vi "Main.vi"(11 "Module Admin":refnum<class "Delacor_lib_QMH_Module Admin.lvclass">) -> ()   [LabVIEW 2024, in "Hardware Controller.lvlib"]
doc: "This template is based off of the Queued Message Handler design pattern and the Queued Message Handler project template that ships with LabVIEW.\n\nThe main difference is that the queue is private to this module and communication between modules is performed via Broadcast and Request events.\n\nRequest events are wrapped in public API methods and are handled in the Event Handling Loop (EHL) of this VI. Any module can register for Broadcast events sent by this module. The EHL generates messages based on user interface actions.\n\nThe Message Handling Loop (MHL) processes messages generated by the EHL, or by other messages. The messages are string values, so new messages can be added easily to the Message Cases case structure in the MHL. Each message cluster can also provide an optional value for Message Data, which is a variant that can be converted to whatever message-specific data is required.\n_____\nBased on DQMH Project Template 7.0.0.1280."
uses:
  Hardware Controller.lvlib
  <vilib>/Delacor/Delacor QMH/Libraries/Module Admin_class/Delacor_lib_QMH_Module Admin.lvclass
  Module Data--cluster.ctl
  <vilib>/Delacor/Delacor QMH/Libraries/Message Queue_class/Delacor_lib_QMH_Message Queue.lvclass/Delacor_lib_QMH_Message Queue.ctl
  Stop Argument--cluster.ctl
  <vilib>/Delacor/Delacor QMH/Libraries/Module Admin_class/Delacor_lib_QMH_Module Admin.lvclass/Delacor_lib_QMH_Module Admin.ctl
  <vilib>/Utility/miscctls.llb/LVPointTypeDef.ctl
  <vilib>/Delacor/Delacor QMH/Libraries/Message Queue_class/Delacor_lib_QMH_Enqueue Message (Single).vi
  <vilib>/Delacor/Delacor QMH/Libraries/Module Admin_class/Delacor_lib_QMH_Get External Launch.vi
  <vilib>/Delacor/Delacor QMH/Libraries/Message Queue_class/Delacor_lib_QMH_Message Queue.lvclass
panel:
  out "System State":map{string, dbl}(c390)
  out "error out":errorcluster
  out "Status":string
  in  "Simulate MHL Error":bool
  in  "Simulate EHL Error":bool
  # "This template is for the DQMH framework. See the block diagram for more information on how to use this template."
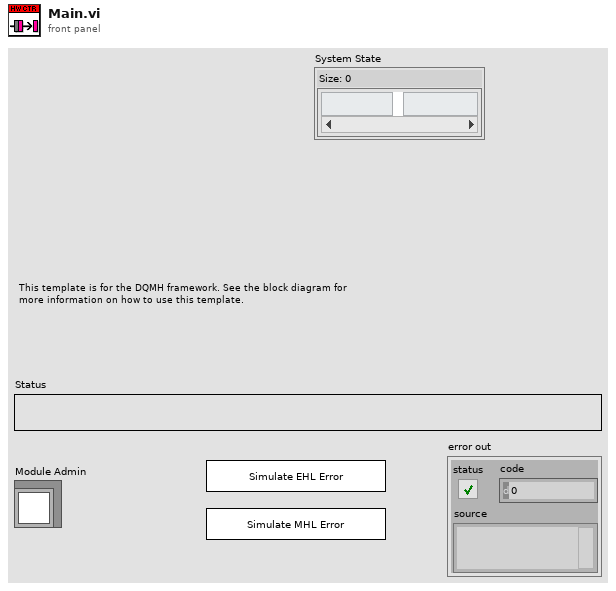
[diagram p1: front panel]
types:
  T1 = typedef "Hardware Controller.lvlib/Request Events--cluster.ctl" = cluster{"Stop Module":refnum<user-event>, "Show Panel":refnum<user-event>, "Hide Panel":refnum<user-event>, "Get Module Execution Status":refnum<user-event>, "Show Diagram":refnum<user-event>, "Private":cluster{"Start System State Broadcast Helper Loop":refnum<user-event>}}
  T2 = typedef "Hardware Controller.lvlib/Module Data--cluster.ctl" = cluster{"Status":string, "System State":map{string, dbl}}
  T3 = enum32{"invalid lock state", "Not Locked", "Locked (No Password)", "Password-protected"}
  T4 = typedef "Hardware Controller.lvlib/Stop Argument--cluster.ctl" = cluster{"Origin":string, "Exit via Stop Module Req?":bool, "Wait for Module to stop?":bool}
  T5 = typedef "LVPointTypeDef.ctl" = cluster{"Horizontal":i16, "Vertical":i16}
  T6 = enum32{"Invalid", "Standard", "Closed", "Hidden", "Minimized", "Maximized"}
  T7 = typedef "EtherCAT Configuration.ctl" = cluster{"ENI File":path, "Drives":cluster{"Drive Key":string, "Read Variables":cluster{"Name":string, "Index":u16, "Bit":u8, "Type":string}[], "Write Variables":cluster{"Name":string, "Index":u16}[]}[]}
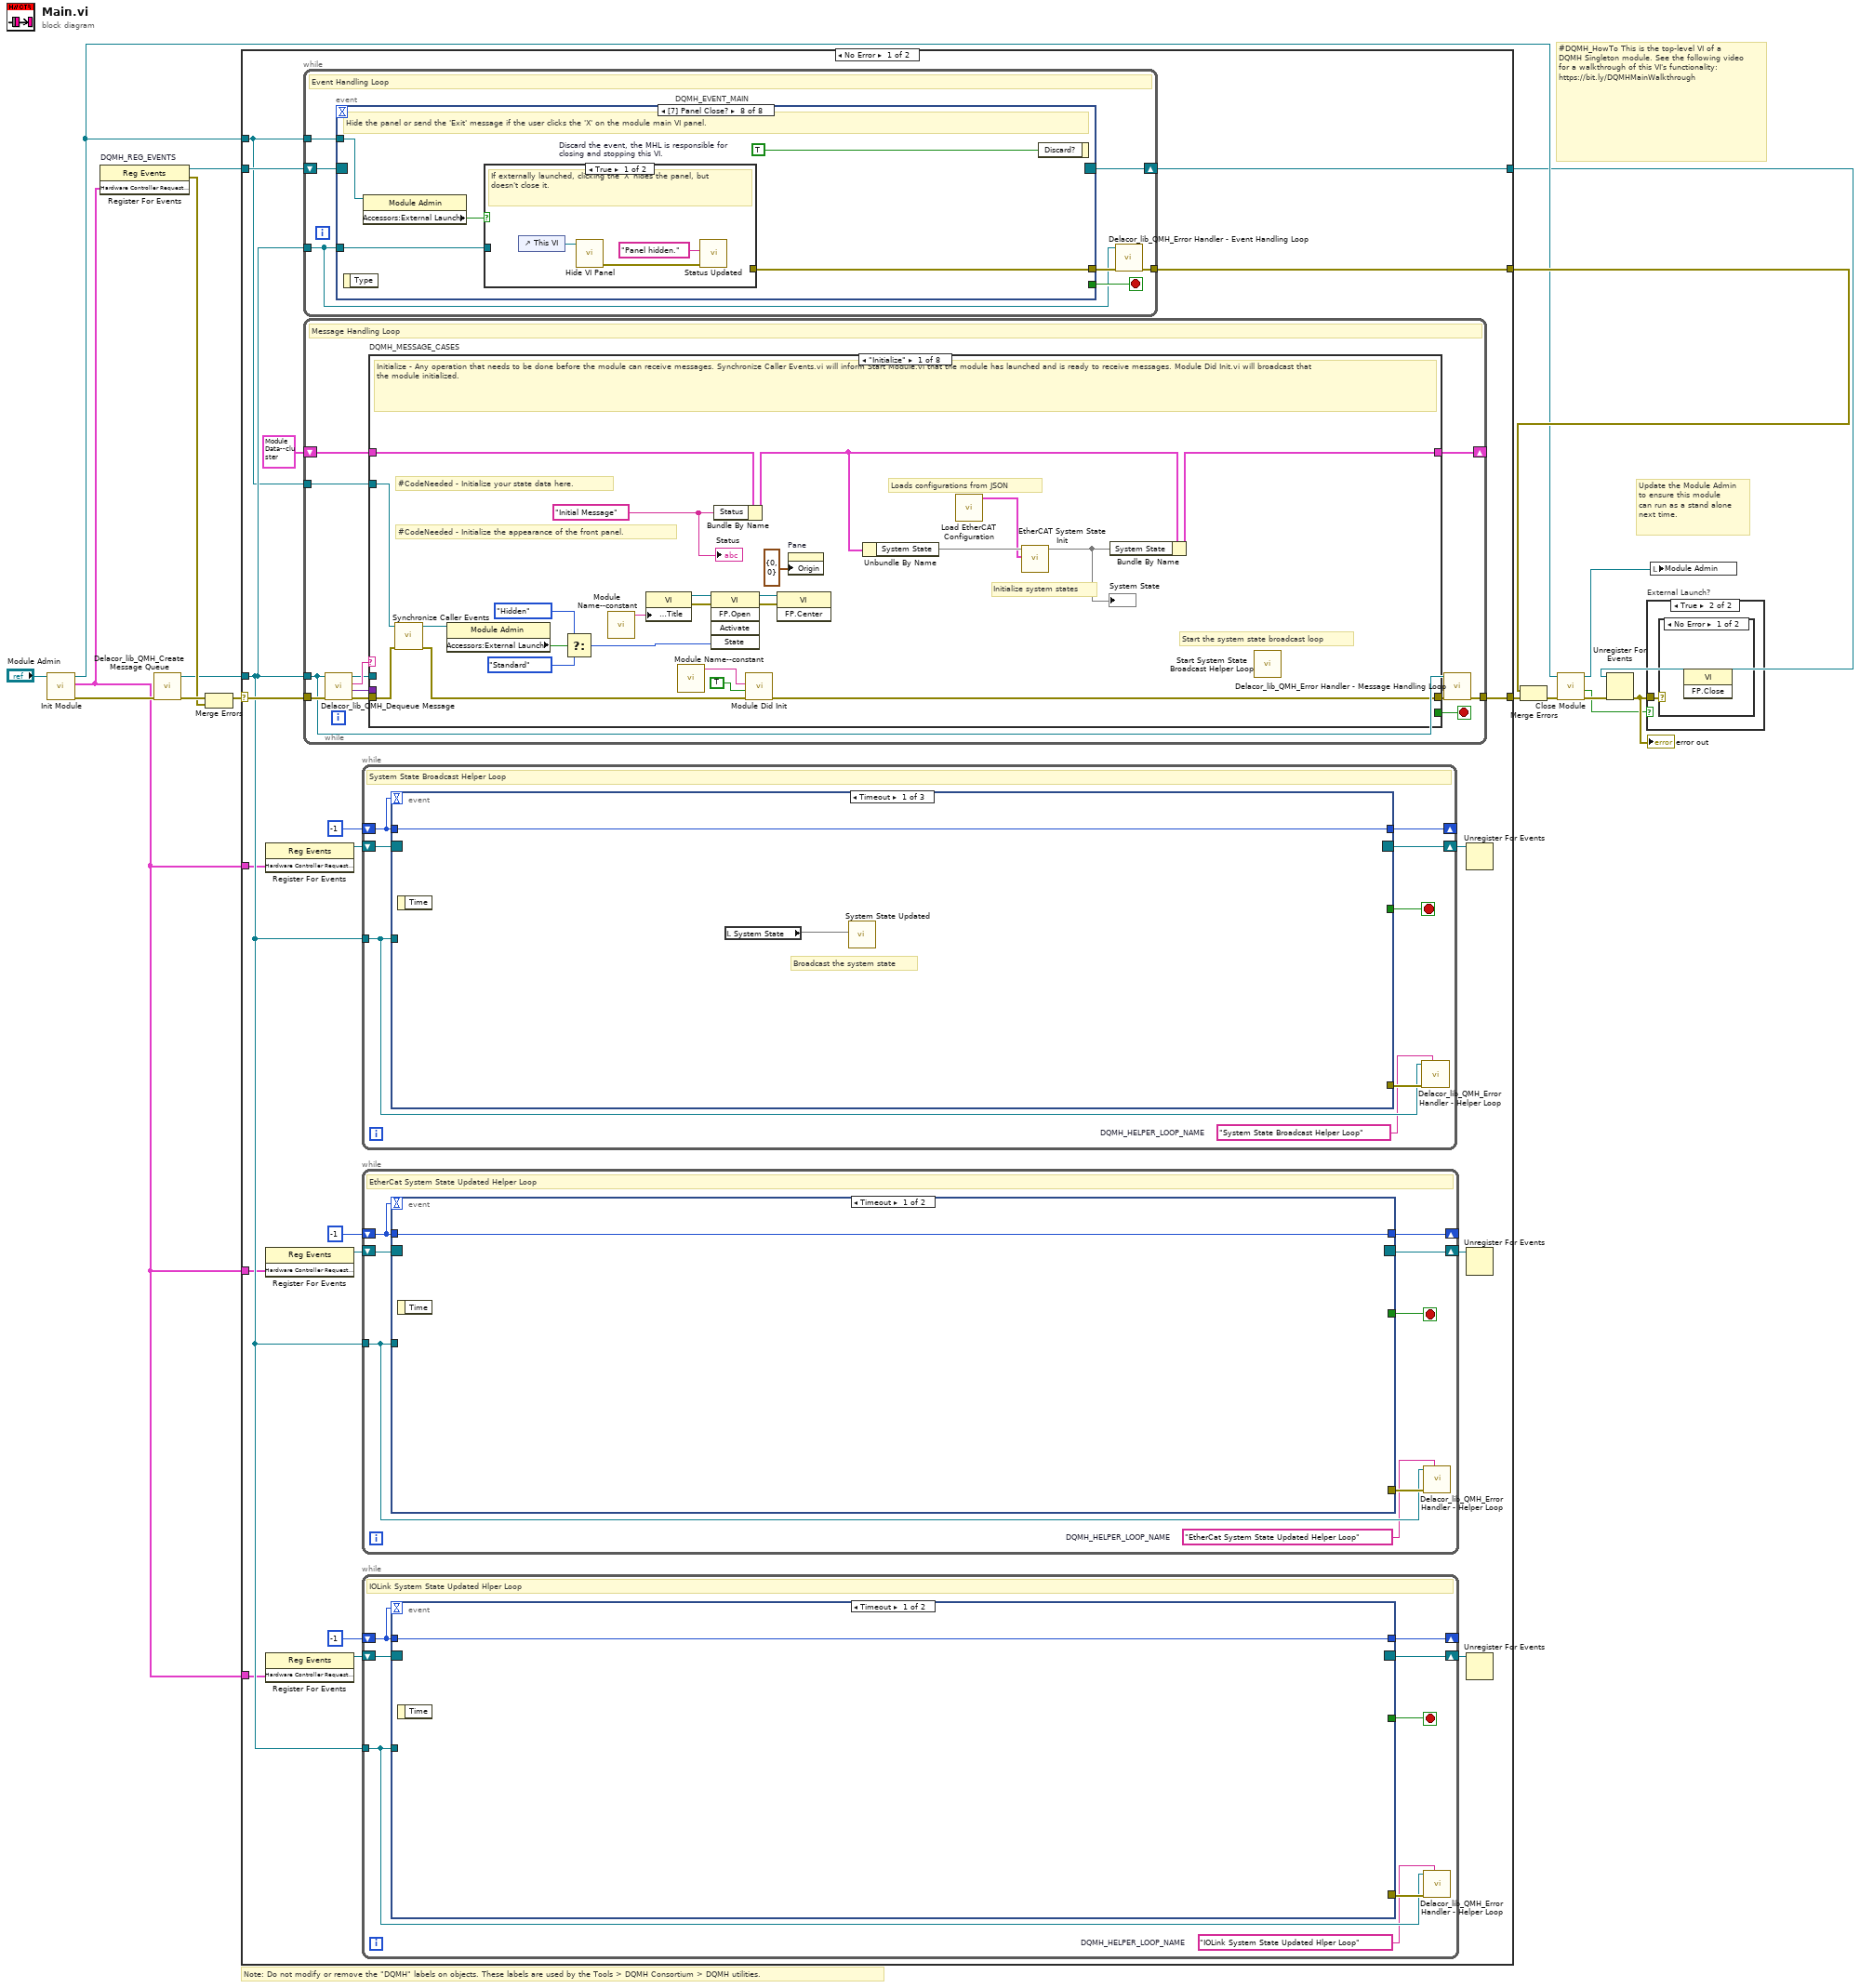
[diagram p0: block diagram]
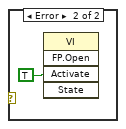
[diagram p3: hidden frame]
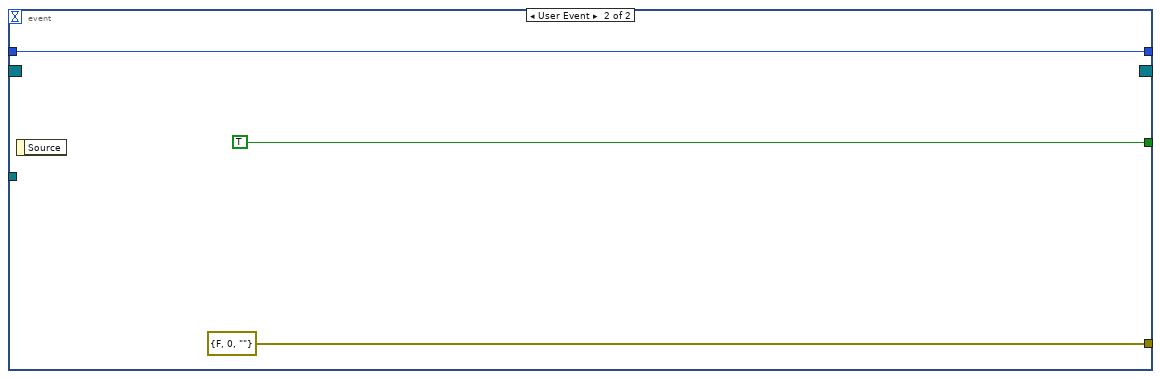
[diagram p4: hidden frame]
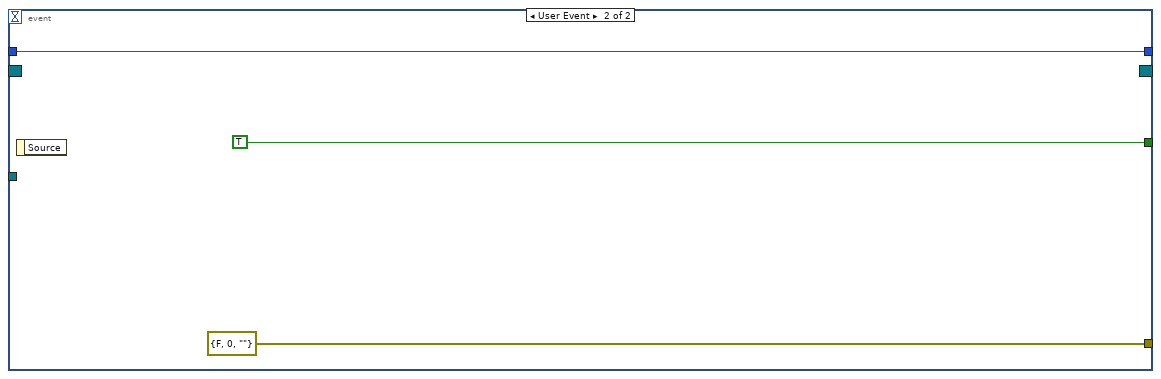
[diagram p5: hidden frame]
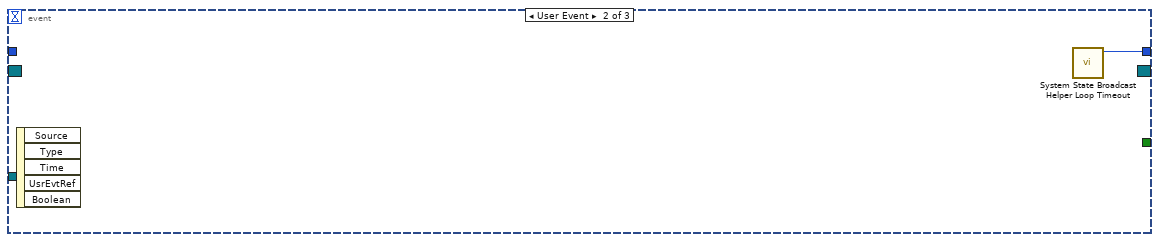
[diagram p6: hidden frame]
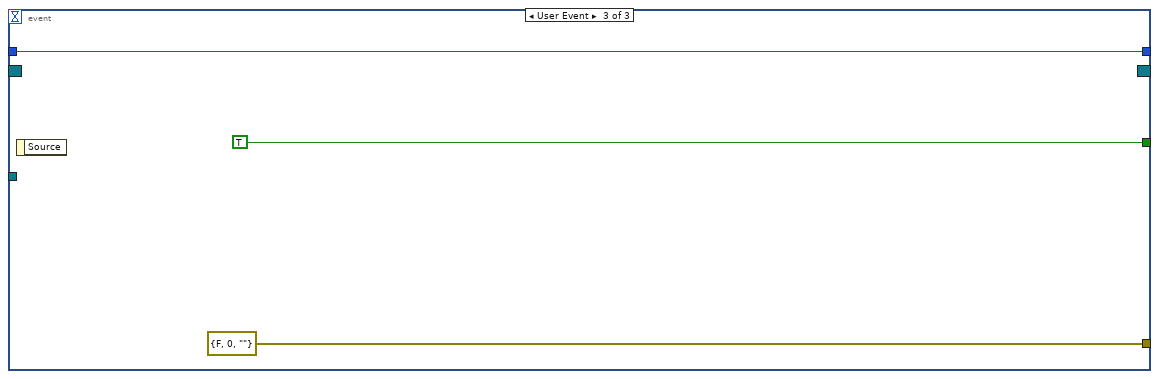
[diagram p7: hidden frame]
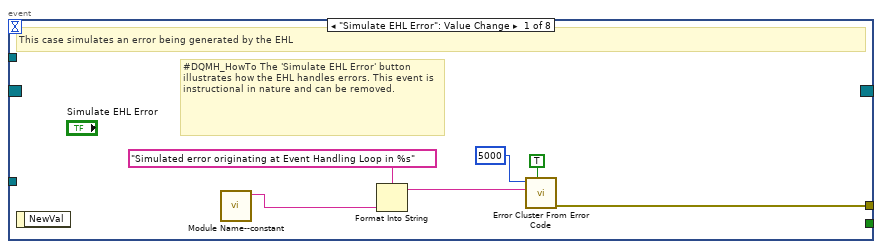
[diagram p8: hidden frame]
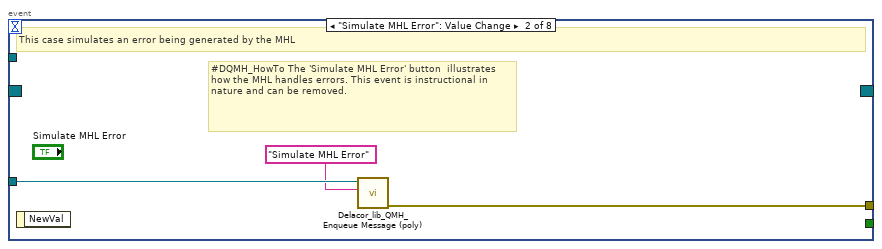
[diagram p9: hidden frame]
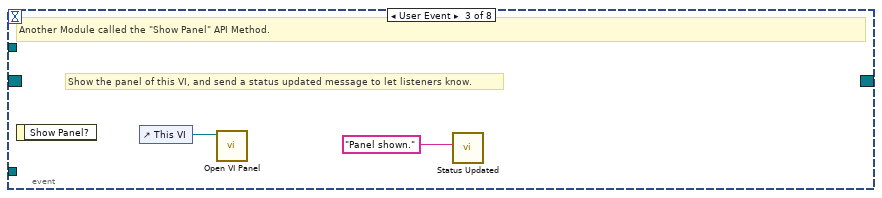
[diagram p10: hidden frame]
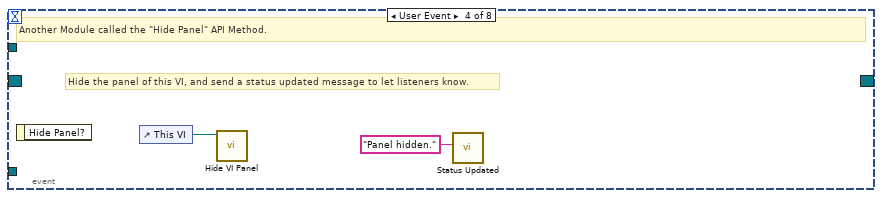
[diagram p11: hidden frame]
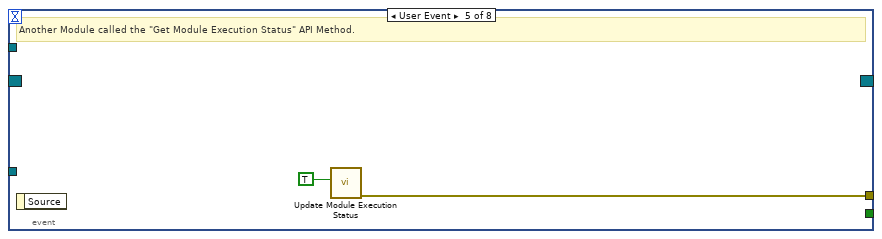
[diagram p12: hidden frame]
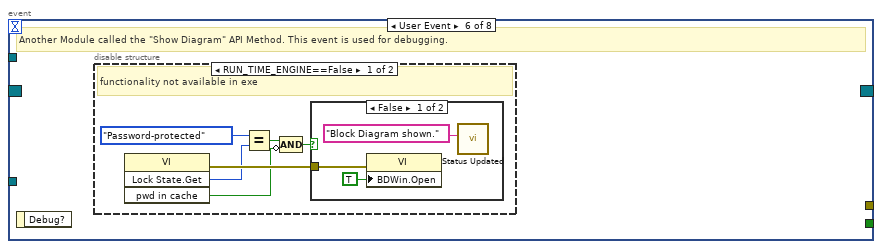
[diagram p13: hidden frame]
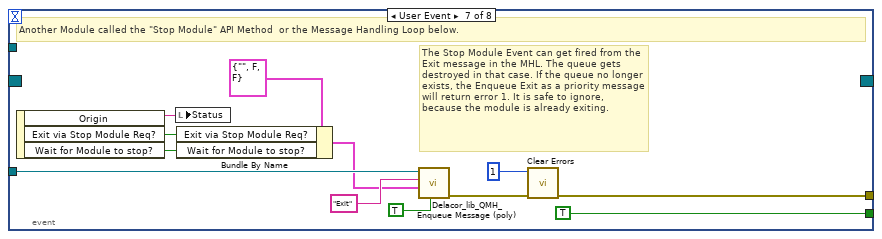
[diagram p16: hidden frame]
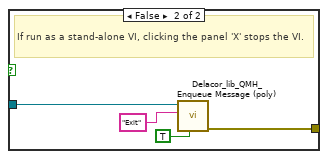
[diagram p17: hidden frame]
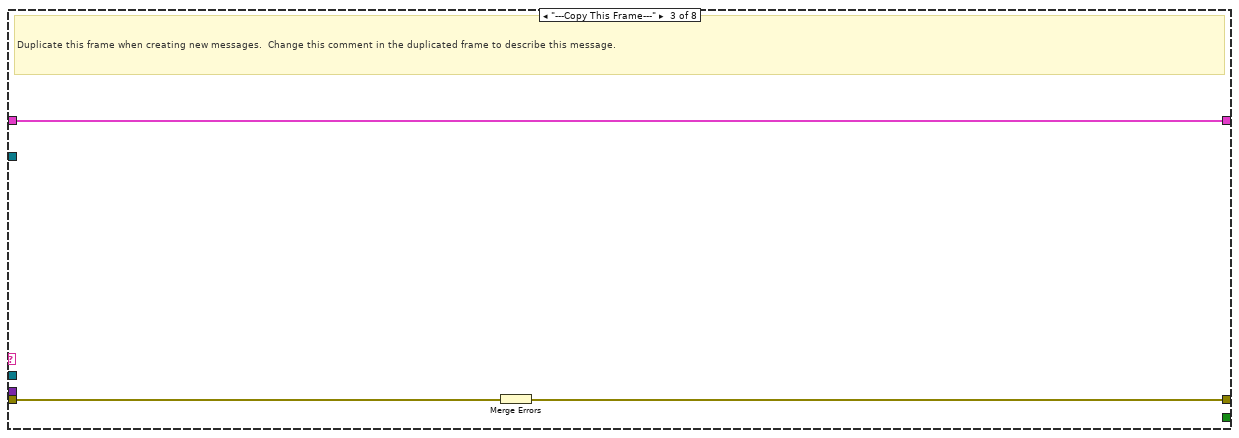
[diagram p19: hidden frame]
diagram:
  # "#DQMH_HowTo This is the top-level VI of a DQMH Singleton module. See the following video for a walkthrough of this VI's functionality: https://bit.ly/DQMHMainWalkthrough"
  # "Note: Do not modify or remove the \"DQMH\" labels on objects. These labels are used by the Tools > DQMH Consortium > DQMH utilities."
  # "Update the Module Admin to ensure this module can run as a stand alone next time."
  n1 = call "Init Module.vi"("Singleton Module Admin in"="Module Admin") -> ("error out"=w16:errorcluster, "Hardware Controller Request Events"=w1:T1, "Singleton Module Admin out"=w8:refnum<class "Delacor_lib_QMH_Module Admin.lvclass">)  [unwired: 8 in]
  n2 = register-events "DQMH_REG_EVENTS"(w1) -> (reference out=w6:refnum<event-registration>, error out=w9:errorcluster)  [unwired: 2 in]
  n3 = call <vilib>:"Delacor_lib_QMH_Create Message Queue.vi"("error in"=w16) -> ("error out"=w11:errorcluster, "Message Queue"=w5:refnum<class "Delacor_lib_QMH_Message Queue.lvclass">)  [unwired: 9 in]
  n4 = Merge Errors(w11, w9) -> (w10:errorcluster)
  n5 = case shown="No Error" w10 {
    selector: w10 -> [w35 w232]
    tunnel: [w37 w231] -> w17
    tunnel: [w34 w230] -> w7
    tunnel: w6 -> [w32 w230]
    tunnel: w5 -> [w31 w225]
    tunnel: [w36 _] -> w14
    tunnel: w8 -> [w30 w226]
    tunnel: w1 -> [w29 _]
    tunnel: w1 -> [w25 _]
    tunnel: w1 -> [w21 _]
    frame No Error {
      n6 = register-events ("DQMH_HELPER_REGFOREVENTS")(w29) -> (reference out=w27:refnum<event-registration>)  [unwired: 2 in, 1 out]
      n7 = register-events ("DQMH_HELPER_REGFOREVENTS")(w25) -> (reference out=w23:refnum<event-registration>)  [unwired: 2 in, 1 out]
      n8 = register-events ("DQMH_HELPER_REGFOREVENTS")(w21) -> (reference out=w19:refnum<event-registration>)  [unwired: 2 in, 1 out]
      n9 = while {
        tunnel: w31 -> [w76]
        shift-right: [w79] -> w34
        shift-left: w32 -> [w80]
        tunnel: [w81] -> w36
        tunnel: w30 -> [w77]
        stop <- w78 stop-if-true
        # "Event Handling Loop"
        n10 = event "DQMH_EVENT_MAIN" shown="[7] Panel Close?" {
          selector: w80 -> [_ _ _ _ _ _ _ _]
          dyn-events: [_ _ _ _ _ _ _ _] -> w79
          timeout: _ -> [_ _ _ _ _ _ _ _]
          tunnel: [_ _ _ _ _ _ TRUE ("Discard?") _] -> w78
          tunnel: w76 -> [_ w90 _ _ _ _ w114 w121]
          tunnel: [w88 w91 _ _ w97 _ w117 w123] -> w82
          tunnel: w77 -> [_ _ _ _ _ _ _ w120]
          event "Simulate EHL Error": Value Change {
            # "#DQMH_HowTo The 'Simulate EHL Error' button  illustrates how the EHL handles errors. This event is instructional in nature and can be removed."
            # "This case simulates an error being generated by the EHL"
            n11 = event-data() -> ()  [unwired: 1 in, 1 out]
            n12 = call "Module Name--constant.vi"() -> ("Module Name"=w85:string)  [unwired: 11 in]
            n13 = Format Into String(format string="Simulated error originating at Event Handling Loop in %s", w85) -> (resulting string=w86:string)  [unwired: 2 in, 1 out]
            n14 = call <vilib>:"Error Cluster From Error Code.vi"("show call chain? (False)"=TRUE, "error message (\"\")"=w86, "error code (0)"=5000) -> ("error out"=w88:errorcluster)  [unwired: 6 in]
          }
          event "Simulate MHL Error": Value Change {
            # "#DQMH_HowTo The 'Simulate MHL Error' button  illustrates how the MHL handles errors. This event is instructional in nature and can be removed."
            # "This case simulates an error being generated by the MHL"
            n15 = event-data() -> ()  [unwired: 1 in, 1 out]
            n16 = call-poly <vilib>:"Delacor_lib_QMH_Enqueue Message (poly).vi"("Message"="Simulate MHL Error", "Message Queue in"=w90) -> ("error out"=w91:errorcluster)  [unwired: 8 in, 1 out]
          }
          event User Event {
            # "Show the panel of this VI, and send a status updated message to let listeners know."
            # "Another Module called the \"Show Panel\" API Method."
            n17 = event-data() -> ()  [unwired: 1 in, 1 out]
            n18 = control-ref of="This VI"() -> (w93:refnum<vi>)
            n19 = call "Open VI Panel.vi"("VI"=w93) -> ()  [unwired: 10 in, 1 out]
            n20 = call "Status Updated.vi"("Status"="Panel shown." ("format string")) -> ()  [unwired: 10 in, 1 out]
          }
          event User Event {
            # "Hide the panel of this VI, and send a status updated message to let listeners know."
            # "Another Module called the \"Hide Panel\" API Method."
            n21 = event-data() -> ()  [unwired: 1 in, 1 out]
            n22 = control-ref of="This VI"() -> (w95:refnum<vi>)
            n23 = call "Hide VI Panel.vi"("VI"=w95) -> ()  [unwired: 10 in, 1 out]
            n24 = call "Status Updated.vi"("Status"="Panel hidden." ("format string")) -> ()  [unwired: 10 in, 1 out]
          }
          event User Event {
            # "Another Module called the \"Get Module Execution Status\" API Method."
            n25 = event-data() -> ()  [unwired: 1 in, 1 out]
            n26 = call "Update Module Execution Status.vi"("Running?"=TRUE) -> ("error out"=w97:errorcluster)  [unwired: 10 in]
          }
          event User Event {
            # "Another Module called the \"Show Diagram\" API Method. This event is used for debugging."
            n27 = event-data() -> ()  [unwired: 1 in, 1 out]
            n28 = disable-structure shown="RUN_TIME_ENGINE==False" {
              frame condition #0 (active) {
                # "functionality not available in exe"
                n29 = invoke class="VI" method="Lock State.Get"() -> (error out=w103:errorcluster, "Get Lock State"=w102:T3, "pwd in cache"=w99:bool)  [unwired: 4 in, 1 out]
                n30 = Equal?(x=T3."Password-protected", y=w102) -> (x = y?=w100:bool)
                n31 = Compound Arithmetic op=AND(w100, invert w99) -> (w98:bool)
                n32 = case shown="False" w98 {
                  tunnel: w103 -> [w106 _]
                  frame False {
                    n33 = property class="VI"(error in=w106, "BDWin.Open"=TRUE ("Block Diagram Window:Open")) -> ()  [unwired: 1 in, 2 out]
                    n34 = call "Status Updated.vi"("Status"="Block Diagram shown." ("format string")) -> ()  [unwired: 10 in, 1 out]
                  }
                  frame True {
                    # "Password-protected VI, and the password is not in the cache. Do not show the diagram."
                  }
                }
              }
              frame condition #1 {
              }
            }
          }
          event User Event {
            # "The Stop Module Event can get fired from the Exit message in the MHL. The queue gets destroyed in that case. If the queue no longer exists, the Enqueue Exit as a priority message will return error 1. It is safe to ignore, because the module is already exiting."
            # "Another Module called the \"Stop Module\" API Method  or the Message Handling Loop below."
            n35 = event-data() -> ("Origin"=w113:string, "Exit via Stop Module Req?"=w109:bool, "Wait for Module to stop?"=w108:bool)  [unwired: 1 in]
            n36 = local write "Status"(w113) -> ()
            n37 = Bundle By Name(cluster=T4 {"Origin"="", "Exit via Stop Module Req?"=FALSE, "Wait for Module to stop?"=FALSE} ("Stop Argument"), "Exit via Stop Module Req?"=w109, "Wait for Module to stop?"=w108) -> (w107:T4)
            n38 = call-poly <vilib>:"Delacor_lib_QMH_Enqueue Message (poly).vi"("Priority Message? (F)"=TRUE, "Message Data"=w107, "Message"="Exit", "Message Queue in"=w114) -> ("error out"=w118:errorcluster)  [unwired: 6 in, 1 out]
            n39 = call <vilib>:"Clear Errors.vi"("error in (no error)"=w118, "specific error code to clear (0: all)"=1) -> ("error out"=w117:errorcluster)  [unwired: 4 in, 1 out]
          }
          event Panel Close? {
            w122 = TRUE  # Discard the event, the MHL is responsible for closing and stopping this VI.
            # "Hide the panel or send the 'Exit' message if the user clicks the 'X' on the module main VI panel."
            n40 = event-data() -> ()  [unwired: 1 in, 1 out]
            n41 = property class="Module Admin"(reference=w120) -> ("Accessors:External Launch"=w119:bool)  [unwired: 1 in, 2 out]
            n42 = case shown="True" w119 {
              tunnel: w121 -> [_ w129]
              tunnel: [_ w130] -> w123
              frame True {
                # "If externally launched, clicking the 'X' hides the panel, but doesn't close it."
                n43 = control-ref of="This VI"() -> (w126:refnum<vi>)
                n44 = call "Hide VI Panel.vi"("VI"=w126) -> ("error out"=w124:errorcluster)  [unwired: 10 in]
                n45 = call "Status Updated.vi"("error in"=w124, "Status"="Panel hidden." ("format string")) -> ()  [unwired: 9 in, 1 out]
              }
              frame False {
                # "If run as a stand-alone VI, clicking the panel 'X' stops the VI."
                n46 = call-poly <vilib>:"Delacor_lib_QMH_Enqueue Message (poly).vi"("Priority Message? (F)"=TRUE, "Message"="Exit", "Message Queue in"=w129) -> ("error out"=w130:errorcluster)  [unwired: 7 in, 1 out]
              }
            }
            n47 = event-data("Discard?"=w122) -> ()  [unwired: 1 in, 1 out]
          }
        }
        n48 = call-dynamic "Delacor_lib_QMH_Error Handler - Event Handling Loop.vi"("error in"=w82, "Message Queue in"=w76) -> ("dup error in"=w81:errorcluster)  [unwired: 8 in, 1 out]
      }
      n49 = while {
        tunnel: w31 -> [w131]
        shift-right: [w137] -> _
        shift-left: T2 {"Status"="", "System State"={}} ("Data Cluster") -> [w138]
        tunnel: w35 -> [w141]
        tunnel: [w139] -> w37
        tunnel: w30 -> [w132]
        stop <- w136 stop-if-true
        # "Message Handling Loop"
        n50 = call-dynamic "Delacor_lib_QMH_Dequeue Message.vi"("error in"=w141, "Message Queue in"=w131) -> ("error out"=w140:errorcluster, "Message Data"=w134:variant, "Message"=w135:string, "Message Queue out"=w133:refnum<class "Delacor_lib_QMH_Message Queue.lvclass">)  [unwired: 6 in]
        n51 = case "DQMH_MESSAGE_CASES" shown="\"Initialize\"" w135 {
          selector: w135 -> [_ _ _ _ _ _ _ w220]
          tunnel: w133 -> [_ _ _ _ _ w186 w208 _]
          tunnel: w140 -> [w164 w168 w171 w173 w182 w193 w214 w223]
          tunnel: [w162 w168 w170 w173 w181 w189 w209 w224] -> w142
          tunnel: w138 -> [w153 w167 w169 w172 w179 w188 w207 w221]
          tunnel: [w144 w167 w169 w172 w179 w188 w207 w221] -> w137
          tunnel: [_ _ _ _ _ _ w206 _] -> w136
          tunnel: w134 -> [_ _ _ _ _ w187 w205 _]
          tunnel: w132 -> [w154 _ _ _ _ w185 w200 _]
          frame "Initialize" {
            w149 = "Initial Message" ("Initial Message")
            # "Start the system state broadcast loop"
            # "Initialize system states"
            # "Loads configurations from JSON"
            # "#CodeNeeded - Initialize the appearance of the front panel."
            # "#CodeNeeded - Initialize your state data here."
            # "Initialize - Any operation that needs to be done before the module can receive messages. Synchronize Caller Events.vi will inform Start Module.vi that the module has launched and is ready to receive messages. Module Did Init.vi will broadcast that the module initialized."
            n52 = call "Synchronize Caller Events.vi"("error in"=w164, "Singleton Module Admin in"=w154) -> ("error out"=w163:errorcluster, "Singleton Module Admin out"=w150:refnum<class "Delacor_lib_QMH_Module Admin.lvclass">)  [unwired: 8 in]
            n53 = property class="Module Admin"(reference=w150) -> ("Accessors:External Launch"=w158:bool)  [unwired: 1 in, 2 out]
            n54 = Select(t=T6."Hidden" ("State"), s=w158, f=T6."Standard" ("State")) -> (s? t:f=w155:T6)
            n55 = call "Module Name--constant.vi"() -> ("Module Name"=w161:string)  [unwired: 11 in]
            n56 = property class="VI"("Front Panel.Title"=w161) -> (reference out=w160:refnum<vi>, error out=w166:errorcluster)  [unwired: 2 in]
            n57 = call "Module Name--constant.vi"() -> ("Module Name"=w151:string)  [unwired: 11 in]
            n58 = invoke class="VI" method="FP.Open"(reference=w160, error in=w166, "State"=w155) -> (reference out=w159:refnum<vi>, error out=w165:errorcluster)  [unwired: 2 in, 3 out]
            n59 = Bundle By Name(cluster=w153, "Status"=w149) -> (w147:T2)
            n60 = call "Module Did Init.vi"("error in"=w163, "Initialized?"=TRUE, "Origin"=w151) -> ("error out"=w162:errorcluster)  [unwired: 8 in]
            n61 = invoke class="VI" method="FP.Center"(reference=w159, error in=w165) -> ()  [unwired: 1 in, 3 out]
            n62 = property on="Pane" class="Pane"("Origin"=T5 {"Horizontal"=0, "Vertical"=0}) -> ()  [unwired: 2 in, 2 out]
            n63 = Unbundle By Name(w147) -> ("System State"=w146:map{string, dbl})
            n64 = call "Load EtherCAT Configuration.vi"() -> ("Setup"=w145:T7)  [unwired: 11 in]
            n65 = call "EtherCAT System State Init.vi"("Setup"=w145, "System State"=w146) -> ("System State Out"=w143:map{string, dbl})  [unwired: 9 in]
            "System State" <- w143
            n66 = Bundle By Name(cluster=w147, "System State"=w143) -> (w144:T2)
            n67 = call "Start System State Broadcast Helper Loop.vi"() -> ()  [unwired: 11 in, 1 out]
            "Status" <- w149
          }
          frame "---Module Specific---" {
            # "Separator -- The following cases handle messages specific to this Module."
          }
          frame "---Copy This Frame---" {
            # "Duplicate this frame when creating new messages.  Change this comment in the duplicated frame to describe this message."
            n68 = Merge Errors(w171) -> (w170:errorcluster)
          }
          frame "---Exit and Error Handling---" {
            # "Separator - The following cases handle errors and exit messages."
          }
          frame "Simulate MHL Error" {
            # "#DQMH_HowTo The 'Simulate MHL Error' button  illustrates how the MHL handles errors. This event is instructional in nature and can be removed."
            # "Simulate an error occurring at the MHL"
            n69 = call "Module Name--constant.vi"() -> ("Module Name"=w175:string)  [unwired: 11 in]
            n70 = Format Into String(format string="Simulated error originating at Message Handling Loop in %s", w175) -> (resulting string=w176:string)  [unwired: 2 in, 1 out]
            n71 = call <vilib>:"Error Cluster From Error Code.vi"("show call chain? (False)"=TRUE, "error message (\"\")"=w176, "error code (0)"=5001) -> ("error out"=w180:errorcluster)  [unwired: 6 in]
            n72 = Merge Errors(w182, w180) -> (w181:errorcluster)
          }
          frame "Error" {
            # "#CodeRecommended - If the module is running in standalone mode (External Launch = FALSE), this code will pop up an error dialog and call the 'Exit' message if an error occurs. Add more fine-grained error management here."
            # "Error - Check the error message data and respond accordingly. This message is sent by the \"Error Handler\" VIs at the end of each loop in this application."
            n73 = property class="Module Admin"(reference=w185) -> ("Accessors:External Launch"=w184:bool)  [unwired: 1 in, 2 out]
            n74 = Variant To Data(error in=w193, type=errorcluster {"status"=FALSE, "code"=0, "source"=""} ("error constant"), Variant=w187) -> (data=w183:errorcluster, error out=w191:errorcluster)
            n75 = local write "error out"(w183) -> ()
            n76 = call "Error Reported.vi"("Error"=w183) -> ()  [unwired: 10 in, 1 out]
            n77 = case shown="False" w184 {
              tunnel: [w198 _] -> w190
              tunnel: w186 -> [w196 _]
              tunnel: w183 -> [w197 _]
              frame False {
                n78 = disable-structure shown="Default" {
                  disable-tunnel: w197 -> [w199 _]
                  frame condition #0 (active) {
                    # "If the module is running standalone, then pop up an error dialog and call the \"Exit\" message."
                    n79 = call <vilib>:"Simple Error Handler.vi"("error in (no error)"=w199) -> ()  [unwired: 4 in, 5 out]
                  }
                  frame condition #1 {
                    # "To prevent the Simple Error Handler VI from being loaded (e.g. when deploying to a Real-Time target), add the Conditional Disable Symbol \"DQMH_Disable_SEH\" to your project and set it to TRUE."
                  }
                }
                n80 = call-poly <vilib>:"Delacor_lib_QMH_Enqueue Message (poly).vi"("Priority Message? (F)"=TRUE, "Message"="Exit", "Message Queue in"=w196) -> ("error out"=w198:errorcluster)  [unwired: 7 in, 1 out]
              }
              frame True {
                # "If the module was launched externally, calling the Error Reported broadcast VI is the only action performed by the \"Error\" message. The module's caller can then process the error appropriately."
              }
            }
            n81 = Merge Errors(w191, w190) -> (w189:errorcluster)
          }
          frame "Exit" {
            w204 = 91  # 91: not all Exit messages will have an argument
            w206 = TRUE  # Stop the VI
            # "Release the message queue reference"
            # "#CodeNeeded - Add any required cleanup code here."
            # "Exit - Exit the application."
            n82 = Variant To Data(error in=w214, type=T4 {"Origin"="", "Exit via Stop Module Req?"=FALSE, "Wait for Module to stop?"=FALSE} ("Stop Argument"), Variant=w205) -> (data=w202:T4, error out=w211:errorcluster)
            n83 = call <vilib>:"Clear Errors.vi"("error in (no error)"=w211, "specific error code to clear (0: all)"=w204) -> ("error out"=w213:errorcluster)  [unwired: 4 in, 1 out]
            n84 = control-ref of="This VI"() -> (w201:refnum<vi>)
            n85 = call-dynamic "Delacor_lib_QMH_Release Message Queue.vi"("error in"=w213, "Message Queue"=w208) -> ("error out"=w212:errorcluster)  [unwired: 9 in]
            n86 = call "Handle Exit.vi"("Stop Argument"=w202, "Admin in"=w200, "VI reference"=w201) -> ("error out"=w210:errorcluster)  [unwired: 7 in, 1 out]
            n87 = Merge Errors(w212, w210) -> (w209:errorcluster)
            n88 = call "Error Reported.vi"("Error"=w209) -> ()  [unwired: 10 in, 1 out]
          }
          frame Default {
            # "'Default' case only runs if there is a message that isn't defined in any of the other cases.  Output a programming error."
            n89 = call "Module Name--constant.vi"() -> ("Module Name"=w219:string)  [unwired: 11 in]
            n90 = Format Into String(format string="The invalid message string \"%s\" was received in the Message Handling Loop for module \"%s\".", w220, w219) -> (resulting string=w215:string)  [unwired: 2 in, 1 out]
            n91 = call <vilib>:"Error Cluster From Error Code.vi"("show call chain? (False)"=TRUE, "error message (\"\")"=w215, "error code (0)"=1) -> ("error out"=w222:errorcluster)  [unwired: 6 in]
            n92 = Merge Errors(w223, w222) -> (w224:errorcluster)
          }
        }
        n93 = call-dynamic "Delacor_lib_QMH_Error Handler - Message Handling Loop.vi"("error in"=w142, "Message Queue in"=w131) -> ("dup error in"=w139:errorcluster)  [unwired: 8 in, 1 out]
      }
      n94 = while "DQMH_HELPER_LOOP" {
        shift-right: [w69] -> _
        shift-left: -1 -> [w68]
        shift-right: [w66] -> w28
        shift-left: w27 -> [w67]
        tunnel: w31 -> [w63]
        stop <- w65 stop-if-true
        w62 = "System State Broadcast Helper Loop"  # DQMH_HELPER_LOOP_NAME
        # "System State Broadcast Helper Loop"
        n95 = event "DQMH_HELPER_EVENT_STRUCTURE" shown="[0] Timeout" {
          selector: w67 -> [_ _ _]
          dyn-events: [_ _ _] -> w66
          timeout: w68 -> [_ _ _]
          tunnel: w68 -> [w71 _ w75]
          tunnel: [w71 w72 w75] -> w69
          tunnel: [_ _ TRUE] -> w65
          tunnel: [_ _ errorcluster {"status"=FALSE, "code"=0, "source"=""} ("error constant")] -> w64
          tunnel: w63 -> [_ _ _]
          event Timeout {
            # "Broadcast the system state"
            n96 = event-data() -> ()  [unwired: 1 in, 1 out]
            n97 = local read "System State"() -> (w70:map{string, dbl})
            n98 = call "System State Updated.vi"("System State"=w70) -> ()  [unwired: 10 in, 1 out]
          }
          event User Event {
            n99 = event-data() -> ()  [unwired: 1 in, 5 out]
            n100 = call "System State Broadcast Helper Loop Timeout.vi"() -> ("timeout"=w72:i32)  [unwired: 11 in]
          }
          event User Event {
            n101 = event-data() -> ()  [unwired: 1 in, 1 out]
          }
        }
        n102 = call-dynamic "Delacor_lib_QMH_Error Handler - Helper Loop.vi"("Error Debug"=w62, "error in"=w64, "Message Queue in"=w63) -> ()  [unwired: 7 in, 2 out]
      }
      n103 = while "DQMH_HELPER_LOOP" {
        shift-right: [w57] -> _
        shift-left: -1 -> [w56]
        shift-right: [w54] -> w24
        shift-left: w23 -> [w55]
        tunnel: w31 -> [w51]
        stop <- w53 stop-if-true
        w50 = "EtherCat System State Updated Helper Loop"  # DQMH_HELPER_LOOP_NAME
        # "EtherCat System State Updated Helper Loop"
        n104 = event "DQMH_HELPER_EVENT_STRUCTURE" shown="[0] Timeout" {
          selector: w55 -> [_ _]
          dyn-events: [_ _] -> w54
          timeout: w56 -> [_ _]
          tunnel: w56 -> [w58 w61]
          tunnel: [w58 w61] -> w57
          tunnel: [_ TRUE] -> w53
          tunnel: [_ errorcluster {"status"=FALSE, "code"=0, "source"=""} ("error constant")] -> w52
          tunnel: w51 -> [_ _]
          event Timeout {
            n105 = event-data() -> ()  [unwired: 1 in, 1 out]
          }
          event User Event {
            n106 = event-data() -> ()  [unwired: 1 in, 1 out]
          }
        }
        n107 = call-dynamic "Delacor_lib_QMH_Error Handler - Helper Loop.vi"("Error Debug"=w50, "error in"=w52, "Message Queue in"=w51) -> ()  [unwired: 7 in, 2 out]
      }
      n108 = while "DQMH_HELPER_LOOP" {
        shift-right: [w45] -> _
        shift-left: -1 -> [w44]
        shift-right: [w42] -> w20
        shift-left: w19 -> [w43]
        tunnel: w31 -> [w39]
        stop <- w41 stop-if-true
        w38 = "IOLink System State Updated Hlper Loop"  # DQMH_HELPER_LOOP_NAME
        # "IOLink System State Updated Hlper Loop"
        n109 = event "DQMH_HELPER_EVENT_STRUCTURE" shown="[0] Timeout" {
          selector: w43 -> [_ _]
          dyn-events: [_ _] -> w42
          timeout: w44 -> [_ _]
          tunnel: w44 -> [w46 w49]
          tunnel: [w46 w49] -> w45
          tunnel: [_ TRUE] -> w41
          tunnel: [_ errorcluster {"status"=FALSE, "code"=0, "source"=""} ("error constant")] -> w40
          tunnel: w39 -> [_ _]
          event Timeout {
            n110 = event-data() -> ()  [unwired: 1 in, 1 out]
          }
          event User Event {
            n111 = event-data() -> ()  [unwired: 1 in, 1 out]
          }
        }
        n112 = call-dynamic "Delacor_lib_QMH_Error Handler - Helper Loop.vi"("Error Debug"=w38, "error in"=w40, "Message Queue in"=w39) -> ()  [unwired: 7 in, 2 out]
      }
      n113 = Unregister For Events(event registration refnum=w28) -> ()  [unwired: 1 in, 1 out]
      n114 = Unregister For Events(event registration refnum=w24) -> ()  [unwired: 1 in, 1 out]
      n115 = Unregister For Events(event registration refnum=w20) -> ()  [unwired: 1 in, 1 out]
    }
    frame Error {
      # "Synchronize Caller Events.vi will inform Start Module.vi that the module has launched and will let the code calling Start Module.vi register for broadcasts and would permit the caller receive the broadcast that an error occurred at launch time."
      n116 = call-dynamic "Delacor_lib_QMH_Release Message Queue.vi"("error in"=w232, "Message Queue"=w225) -> ("error out"=w231:errorcluster)  [unwired: 9 in]
      n117 = call "Synchronize Caller Events.vi"("Singleton Module Admin in"=w226) -> ("error out"=w233:errorcluster)  [unwired: 9 in, 1 out]
      n118 = call "Module Name--constant.vi"() -> ("Module Name"=w229:string)  [unwired: 11 in]
      n119 = Format Into String(format string="An error occurred during initialization. %s is no longer running.", w229) -> (resulting string=w227:string)  [unwired: 2 in, 1 out]
      n120 = Merge Errors(w231, w233) -> (w234:errorcluster)
      n121 = call "Error Reported.vi"("Additional Information"=w227, "Error"=w234) -> ()  [unwired: 9 in, 1 out]
    }
  }
  n122 = Merge Errors(w14, w17) -> (w13:errorcluster)
  n123 = call "Close Module.vi"("error in"=w13, "Module Admin in"=w8) -> ("error out"=w15:errorcluster, "External Launch"=w2:bool, "Module Admin out"=w3:refnum<class "Delacor_lib_QMH_Module Admin.lvclass">)  [unwired: 7 in]
  n124 = Unregister For Events(event registration refnum=w7, error in=w15) -> (error out=w12:errorcluster)
  "error out" <- w12
  n125 = case "External Launch?" shown="True" w2 {
    tunnel: w12 -> [_ w235]
    frame False {
    }
    frame True {
      n126 = case shown="No Error" w235 {
        frame No Error {
          n127 = invoke class="VI" method="FP.Close"() -> ()  [unwired: 3 in, 3 out]
        }
        frame Error {
          n128 = invoke class="VI" method="FP.Open"("Activate"=TRUE ("Activate?")) -> ()  [unwired: 4 in, 5 out]
        }
      }
    }
  }
  n129 = local write "Module Admin"(w3) -> ()
